vi "write file to 5071C.vi"(8 "error in (no error)":errorcluster, 11 "VISA resource name":refnum<visa-resource-name>) -> (0 "error out":errorcluster, 3 "VISA resource name out":refnum<visa-resource-name>)   [LabVIEW 2011]
uses:
  Agilent ENA Series/Agilent ENA Series.lvlib
panel:
  in  "网分路径(D:)":string="HXState.STA"
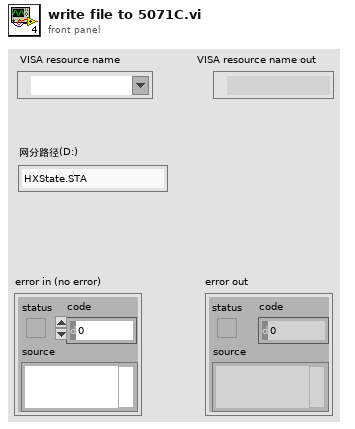
[diagram p1: front panel]
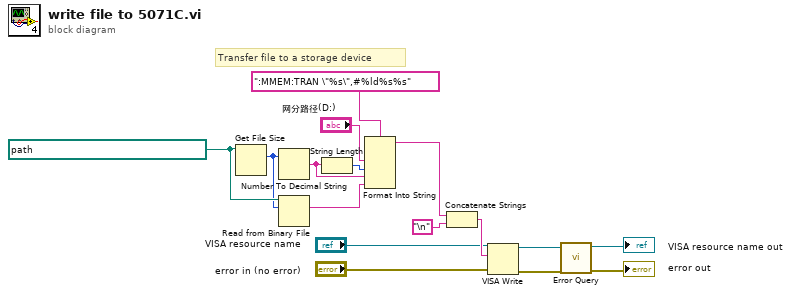
[diagram p0: block diagram]
diagram:
  w5 = path "D:/E5071C校准状态/HXState.STA" ("本机文件")
  # "Transfer file to a storage device"
  n1 = Get File Size(file=w5) -> (size (in bytes)=w3:i64)  [unwired: 1 in, 2 out]
  n2 = Number To Decimal String(number=w3) -> (decimal integer string=w1:string)  [unwired: 1 in]
  n3 = Read from Binary File(10:w3, 11:w5) -> (2:w13:string)  [unwired: 4 in, 3 out]
  n4 = String Length(string=w1) -> (length=w2:i32)
  n5 = Format Into String(format string=":MMEM:TRAN \"%s\",#%ld%s%s", "网分路径(D:)", w2, w1, w13) -> (resulting string=w10:string)  [unwired: 2 in, 1 out]
  n6 = Concatenate Strings(w10, "\n") -> (w12:string)
  n7 = VISA Write(VISA resource name="VISA resource name", write buffer=w12, error in (no error)="error in (no error)") -> (VISA resource name out=w7:refnum<visa-resource-name>, error out=w6:errorcluster)  [unwired: 1 out]
  n8 = call "Error Query.vi"("error in (no error)"=w6, "VISA resource name"=w7) -> ("error out"=→"error out":errorcluster, "VISA resource name out"=→"VISA resource name out":refnum<visa-resource-name>)  [unwired: 6 in, 2 out]
